vi "conectingPythontoLabview.vi"   [LabVIEW 2024]
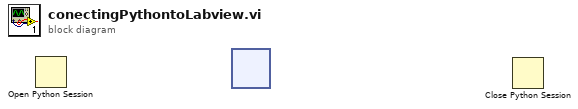
[diagram p0: block diagram]
diagram:
  n1 = Open Python Session() -> ()  [unwired: 3 in, 2 out]
  n2 = node() -> ()  [unwired: 6 in, 4 out]
  n3 = Close Python Session() -> ()  [unwired: 2 in, 1 out]
